vi "Encoder Reset.vi"(0 "Arduino Resource":T1={"VISA resource"="COM11", "Board Type"=enum."Uno", "Connection Type"=enum."USB / Serial", "Bytes Per Packet (15)"=15}, 7 "Encoder Number (0)":u8, 11 "error in":errorcluster) -> (4 "Arduino Resource Out":T1={"VISA resource"="COM11", "Board Type"=enum."Uno", "Connection Type"=enum."USB / Serial", "Bytes Per Packet (15)"=15}, 15 "error out":errorcluster)   [LabVIEW 2012]
doc: "Set encoder value on Arduino to zero.\nArduino Mega 2560 pin pairs to use for encoders (0, 1, 2) are 2 & 3, 18 & 19, 20 & 21.\nArduino Uno only has one pair of pins, 2 & 3 (encoder index 0).\nMust use the custom encoder version of the LIFA firmware."
uses:
  <vilib>/LabVIEW Interface for Arduino/Type Defs/Arduino Resource.ctl
  <vilib>/LabVIEW Interface for Arduino/Type Defs/Board Type.ctl
  <vilib>/LabVIEW Interface for Arduino/LabVIEW Interface for Arduino.lvlib
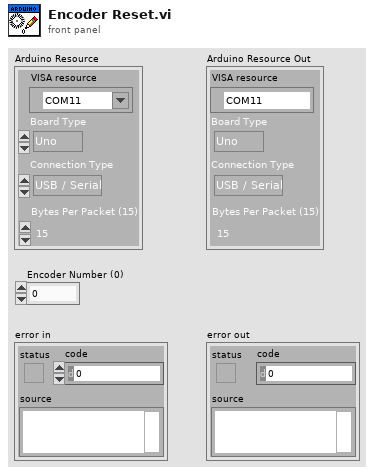
[diagram p1: front panel]
types:
  T1 = typedef "LabVIEW Interface for Arduino.lvlib/Arduino Resource.ctl" = cluster{"VISA resource":refnum<visa-resource-name>, "Board Type":T2, "Connection Type":enum8{"USB / Serial"}, "Bytes Per Packet (15)":u8}
  T2 = typedef "LabVIEW Interface for Arduino.lvlib/Board Type.ctl" = enum16{"Uno", "Dimuelanove w/Atmega 328", "Mega 2560"}
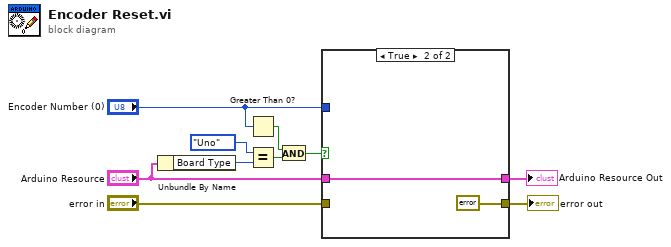
[diagram p0: block diagram]
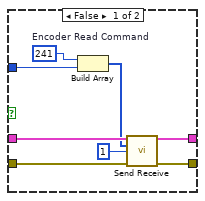
[diagram p2: hidden frame]
diagram:
  n1 = Unbundle By Name("Arduino Resource") -> ("Board Type"=w4:T2)
  n2 = Greater Than 0?(x="Encoder Number (0)") -> (x > 0?=w6:bool)
  n3 = Equal?(x=Board_Type."Uno", y=w4) -> (x = y?=w7:bool)
  n4 = And(x=w6, y=w7) -> (x .and. y?=w1:bool)
  n5 = case shown="True" w1 {
    tunnel: [w18 w19] -> w10
    tunnel: [w17 errorcluster {"status"=TRUE, "code"=0, "source"="Arduino Uno only has one encoder (index 0)."} ("error out")] -> w9
    tunnel: "error in" -> [w16 _]
    tunnel: "Arduino Resource" -> [w15 w19]
    tunnel: "Encoder Number (0)" -> [w12 _]
    frame False {
      w11 = u8 241  # Encoder Read Command
      n6 = Build Array(w11, w12) -> (w13:u8[])
      n7 = call <vilib>:"Send Receive.vi"("Arduino Resource"=w15, "Data"=w13, "Bytes To Read (0)"=u8 1, "error in"=w16) -> ("Arduino Resource"=w18:T1, "error out"=w17:errorcluster)  [unwired: 9 in, 1 out]
    }
    frame True {
    }
  }
  "error out" <- w9
  "Arduino Resource Out" <- w10
